vi "Double Scanner.vi"(6 "error in (no error)":errorcluster, 8 "Range Array":T1[](array[typedef]), 9 "Scanner 2 in":refnum<class "Scanner.lvclass">, 10 "Scanner 1 in":refnum<class "Scanner.lvclass">, 11 "Double Scanner in":refnum<class "Double Scanner.lvclass">) -> (0 "error out":errorcluster, 3 "Double Scanner out":refnum<class "Double Scanner.lvclass">)   [LabVIEW 2017, in "Double Scanner.lvclass"]
uses:
  Double Scanner.lvclass
  Scanner/Range.ctl
  Scanner/Scanner.lvclass
panel:
  in  "Empyty Range":T1
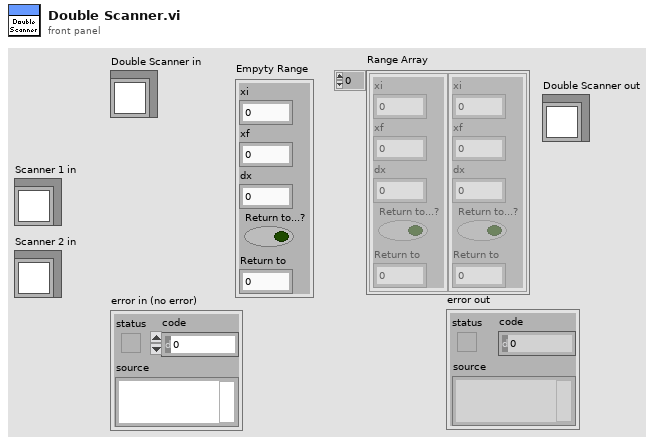
[diagram p1: front panel]
types:
  T1 = typedef "Scanner.lvclass/Range.ctl" = cluster{"xi":dbl, "xf":dbl, "dx":dbl, "Return to...?":bool, "Return to":dbl}
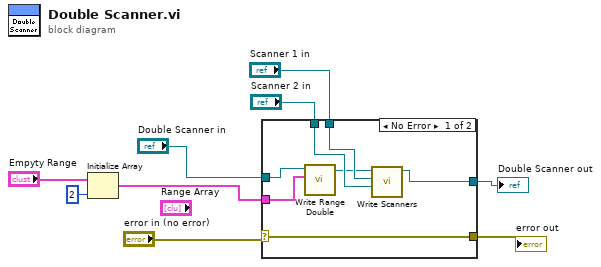
[diagram p0: block diagram]
diagram:
  n1 = Initialize Array("Empyty Range", 2 ("dimension size")) -> (w1:T1[])
  n2 = case shown="No Error" "error in (no error)" {
    selector: "error in (no error)" -> [w16 w18]
    tunnel: [w16 w18] -> w8
    tunnel: "Double Scanner in" -> [w14 w17]
    tunnel: [w13 w17] -> w6
    tunnel: w1 -> [w15 _]
    tunnel: "Scanner 2 in" -> [w12 _]
    tunnel: "Scanner 1 in" -> [w11 _]
    frame No Error {
      n3 = call-dynamic "Write Range Double.vi"("Range Array"=w15, "Double Scanner in"=w14) -> ("Double Scanner out"=w10:refnum<class "Double Scanner.lvclass">)  [unwired: 7 in, 2 out]
      n4 = call "Write Scanners.vi"("Scanner 2 in"=w12, "Scanner 1 in"=w11, "Double Scanner in"=w10) -> ("Double Scanner out"=w13:refnum<class "Double Scanner.lvclass">)  [unwired: 7 in, 1 out]
    }
    frame Error {
    }
  }
  "Double Scanner out" <- w6
  "error out" <- w8
